vi "IncenterTriangle.vi"(6 "C":dbl[](array[numeric]), 8 "error in (no error)":errorcluster, 9 "B":dbl[](array[numeric]), 10 "A":dbl[](array[numeric]), 11 "Utilities in":refnum<class "Utilities.lvclass">) -> (0 "error out":errorcluster, 2 "I":dbl[](array[numeric]), 3 "Utilities out":refnum<class "Utilities.lvclass">)   [LabVIEW 2020, in "Utilities.lvclass"]
uses:
  Utilities.lvclass
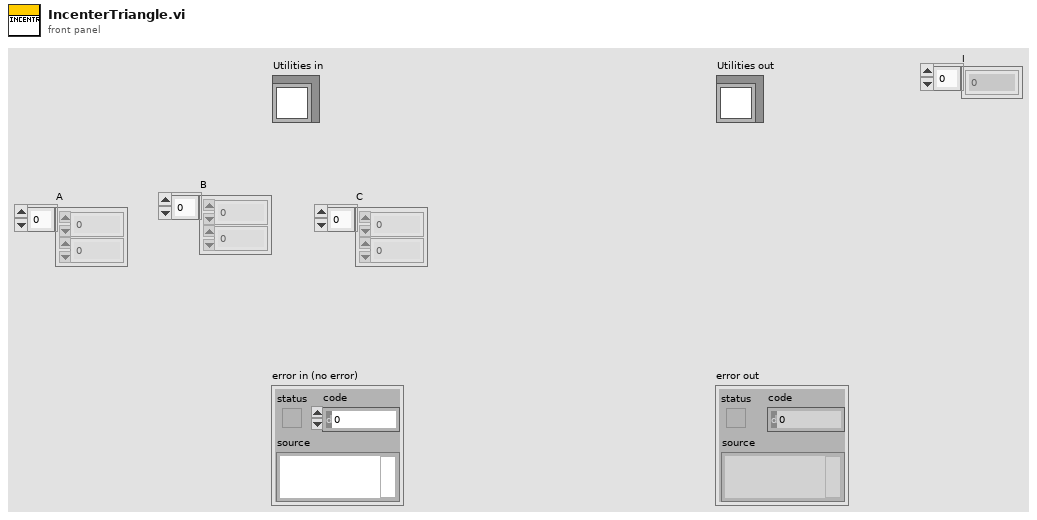
[diagram p1: front panel]
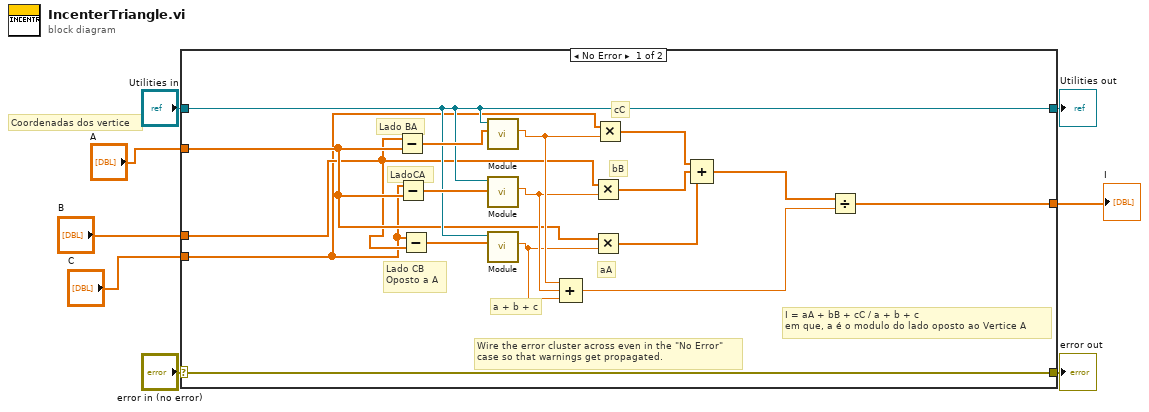
[diagram p0: block diagram]
diagram:
  # "Coordenadas dos vertice"
  n1 = case shown="No Error" "error in (no error)" {
    selector: "error in (no error)" -> [w25 w27]
    tunnel: [w25 w27] -> w7
    tunnel: [w13 w26] -> w5
    tunnel: "Utilities in" -> [w13 w26]
    tunnel: "A" -> [w12 _]
    tunnel: "B" -> [w11 _]
    tunnel: "C" -> [w10 _]
    tunnel: [w9 _] -> w1
    frame No Error {
      # "a + b + c"
      # "bB"
      # "cC"
      # "aA"
      # "I = aA + bB + cC / a + b + c\nem que, a é o modulo do lado oposto ao Vertice A"
      # "Lado CB\nOposto a A"
      # "LadoCA"
      # "Lado BA"
      # "Wire the error cluster across even in the \"No Error\"\ncase so that warnings get propagated."
      n2 = Subtract(x=w11, y=w12) -> (x-y=w16:dbl[])
      n3 = Subtract(x=w10, y=w12) -> (x-y=w15:dbl[])
      n4 = Subtract(x=w10, y=w11) -> (x-y=w14:dbl[])
      n5 = call-dynamic "Module.vi"("2D vector"=w16, "Utilities in"=w13) -> ("Modulo"=w21:dbl)  [unwired: 7 in, 2 out]
      n6 = call-dynamic "Module.vi"("2D vector"=w15, "Utilities in"=w13) -> ("Modulo"=w20:dbl)  [unwired: 7 in, 2 out]
      n7 = call-dynamic "Module.vi"("2D vector"=w14, "Utilities in"=w13) -> ("Modulo"=w19:dbl)  [unwired: 7 in, 2 out]
      n8 = Compound Arithmetic op=ADD(w21, w20, w19) -> (w17:dbl)
      n9 = Multiply(x=w11, y=w20) -> (x*y=w23:dbl[])
      n10 = Multiply(x=w12, y=w19) -> (x*y=w22:dbl[])
      n11 = Multiply(x=w10, y=w21) -> (x*y=w24:dbl[])
      n12 = Compound Arithmetic op=ADD(w24, w23, w22) -> (w18:dbl[])
      n13 = Divide(x=w18, y=w17) -> (x/y=w9:dbl[])
    }
    frame Error {
    }
  }
  "error out" <- w7
  "Utilities out" <- w5
  "I" <- w1
